vi "Load VGC Configuration Settings from XML.vi"(8 "error in (no error)":errorcluster, 11 "Data":T1={"UI References"={"Exit Ref"=refnum, "Save Ref"=refnum, "Export Ref"=refnum, "Acquire Ref"=refnum, "Configure Ref"=refnum, "Graph Ref"=refnum, "Analyze Ref"=refnum, "Status Ref"=refnum, "Snapshot Ref"=refnum, "Start Ref"=refnum}, "Vacuum Graph config"={"Log/Lin"=FALSE, "Show Backing"=FALSE, "Show Chamber"=FALSE}, "VGC50"={"serial settings"={"port"="Inficon_VGC503", "baud rate"=115200}, "device information"={"type"="", "model number"="", "serial number"="", "firmware version"="", "hardware version"=""}, "VGC"=refnum, "Backing SP"={"mode"=2, "thresholds"={"lower"=0.1, "upper"=1.0}, "on"=FALSE}, "Chamber SP"={"mode"=3, "thresholds"={"lower"=1e-05, "upper"=0.0001}, "on"=FALSE}}} {"VGC50"."Chamber SP"."thresholds"."upper" format="%#_5p"; "VGC50"."Chamber SP"."thresholds"."lower" format="%#_5p"; "VGC50"."Chamber SP"."mode" items=["off", "on", "channel 1", "channel 2", "channel 3"]; "VGC50"."Backing SP"."thresholds"."upper" format="%#_5p"; "VGC50"."Backing SP"."thresholds"."lower" format="%#_5p"; "VGC50"."Backing SP"."mode" items=["off", "on", "channel 1", "channel 2", "channel 3"]; "VGC50"."serial settings"."baud rate" items=["9600"=9600, "19200"=19200, "38400"=38400, "57600"=57600, "115200"=115200]}) -> (0 "error out":errorcluster, 3 "User Specified Out":T1={"UI References"={"Exit Ref"=refnum, "Save Ref"=refnum, "Export Ref"=refnum, "Acquire Ref"=refnum, "Configure Ref"=refnum, "Graph Ref"=refnum, "Analyze Ref"=refnum, "Status Ref"=refnum, "Snapshot Ref"=refnum, "Start Ref"=refnum}, "Vacuum Graph config"={"Log/Lin"=FALSE, "Show Backing"=FALSE, "Show Chamber"=FALSE}, "VGC50"={"serial settings"={"port"="Inficon_VGC503", "baud rate"=115200}, "device information"={"type"="", "model number"="", "serial number"="", "firmware version"="", "hardware version"=""}, "VGC"=refnum, "Backing SP"={"mode"=2, "thresholds"={"lower"=0.1, "upper"=1.0}, "on"=FALSE}, "Chamber SP"={"mode"=3, "thresholds"={"lower"=1e-05, "upper"=0.0001}, "on"=FALSE}}} {"VGC50"."Chamber SP"."thresholds"."upper" format="%#_5p"; "VGC50"."Chamber SP"."thresholds"."lower" format="%#_5p"; "VGC50"."Chamber SP"."mode" items=["off", "on", "channel 1", "channel 2", "channel 3"]; "VGC50"."Backing SP"."thresholds"."upper" format="%#_5p"; "VGC50"."Backing SP"."thresholds"."lower" format="%#_5p"; "VGC50"."Backing SP"."mode" items=["off", "on", "channel 1", "channel 2", "channel 3"]; "VGC50"."serial settings"."baud rate" items=["9600"=9600, "19200"=19200, "38400"=38400, "57600"=57600, "115200"=115200]})   [LabVIEW 2024]
doc: "Attempts to load previous user specified settings from an XML file.\n\nThis VI will not generate an error. If a suitable XML file can't be loaded and parsed then it will simply return the default settings."
uses:
  Program Files/National Instruments/LabVIEW 2024/instr.lib/PL Inficon VGC/PL Inficon VGC.lvclass
  <vilib>/Utility/xml.llb/Read From XML File(string).vi
  controls/VGC50.ctl
  controls/Vac Graph Config.ctl
  controls/UI References.ctl
  controls/VGCData.ctl
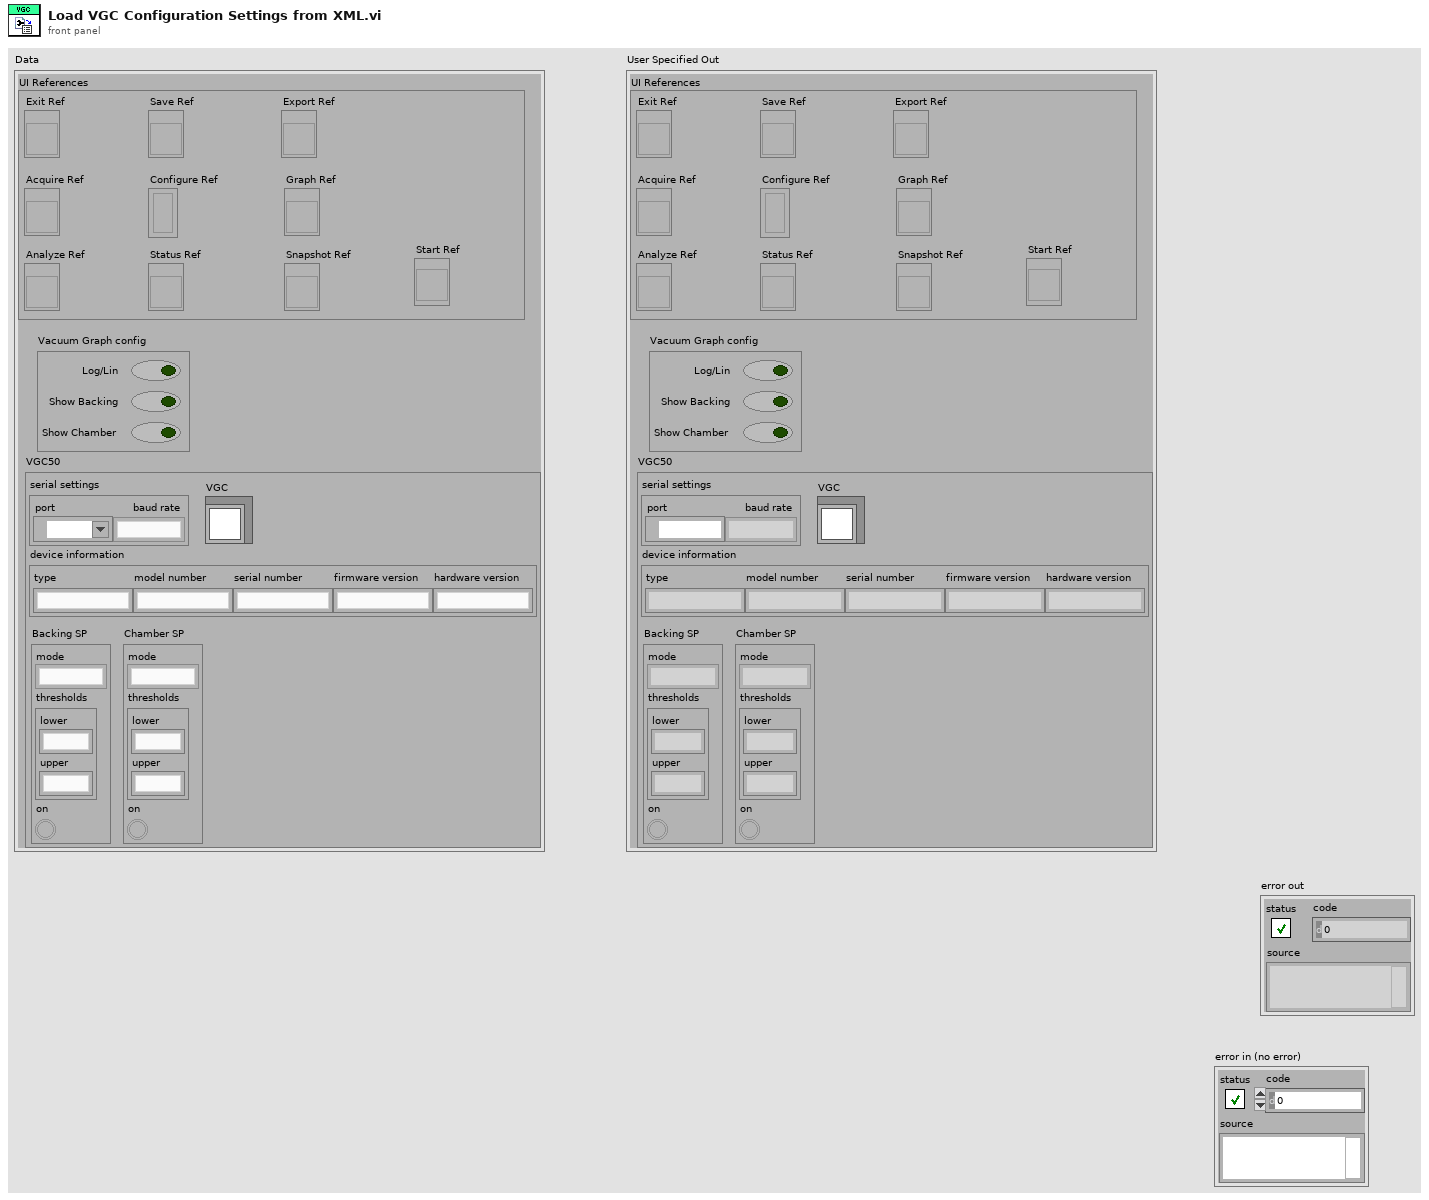
[diagram p1: front panel]
types:
  T1 = typedef "VGCData.ctl" = cluster{"UI References":T2, "Vacuum Graph config":T3, "VGC50":T4}
  T2 = typedef "UI References.ctl" = cluster{"Exit Ref":refnum<vi>, "Save Ref":refnum<vi>, "Export Ref":refnum<vi>, "Acquire Ref":refnum<vi>, "Configure Ref":refnum<vi>, "Graph Ref":refnum<vi>, "Analyze Ref":refnum<vi>, "Status Ref":refnum<vi>, "Snapshot Ref":refnum<vi>, "Start Ref":refnum<vi>}
  T3 = typedef "Vac Graph Config.ctl" = cluster{"Log/Lin":bool, "Show Backing":bool, "Show Chamber":bool}
  T4 = typedef "VGC50.ctl" = cluster{"serial settings":cluster{"port":refnum<visa-resource-name>, "baud rate":u32}, "device information":cluster{"type":string, "model number":string, "serial number":string, "firmware version":string, "hardware version":string}, "VGC":refnum<class "PL Inficon VGC.lvclass">, "Backing SP":cluster{"mode":u16, "thresholds":cluster{"lower":dbl, "upper":dbl}, "on":bool}, "Chamber SP":cluster{"mode":u16, "thresholds":cluster{"lower":dbl, "upper":dbl}, "on":bool}}
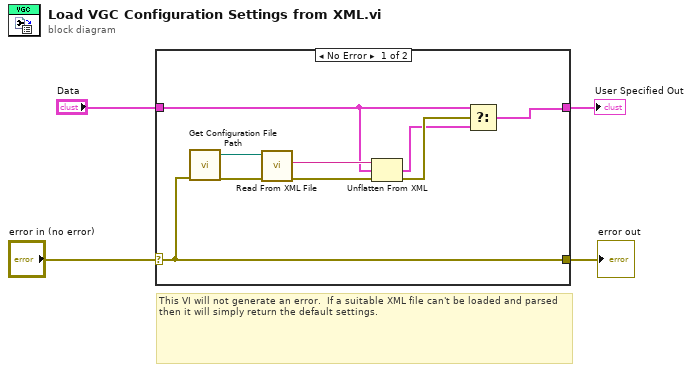
[diagram p0: block diagram]
diagram:
  # "This VI will not generate an error.  If a suitable XML file can't be loaded and parsed then it will simply return the default settings."
  n1 = case shown="No Error" "error in (no error)" {
    selector: "error in (no error)" -> [w10 w15]
    tunnel: [w10 w15] -> w3
    tunnel: "Data" -> [w7 w14]
    tunnel: [w5 w14] -> w1
    frame No Error {
      n2 = call "Get Configuration File Path.vi"("error in (no error)"=w10) -> ("error out"=w12:errorcluster, "XML File Path"=w13:path)  [unwired: 9 in]
      n3 = call-poly <vilib>:"Read From XML File.vi"("error in (no error)"=w12, "XML File Path"=w13) -> ("error out"=w9:errorcluster, "XML Elements"=w11:string)  [unwired: 7 in, 1 out]
      n4 = Unflatten From XML(xml string=w11, type=w7, error in (no error)=w9) -> (value=w6:T1, error out=w8:errorcluster)
      n5 = Select(t=w7, s=w8, f=w6) -> (s? t:f=w5:T1)
    }
    frame Error {
    }
  }
  "error out" <- w3
  "User Specified Out" <- w1
